vi "Build Application and Installer.vi"(10 "Package Version":string, 11 "Path to project":path) -> (0 "error out":errorcluster)   [LabVIEW 2019]
doc: "Builds the Application (EXE) and Installer with <b>Package Version</b> from build specs in <b>Path to project</b>"
uses:
  Build/Typedefs/Build Spec Type--combo.ctl
  <vilib>/AppBuilder/AB_API_Simple/Set Build Specification Version (path).vi
  <vilib>/AppBuilder/AB_API_Simple/Build (path).vi
  Build/Build.lvlib
  <vilib>/AppBuilder/AB_API_Simple/NI_App_Builder_API.lvlib
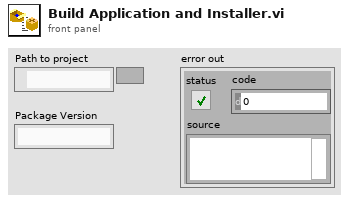
[diagram p1: front panel]
types:
  T1 = typedef "Build.lvlib/Build Spec Type--combo.ctl" = string
  T2 = typedef "Build.lvlib/Build Spec--cluster.ctl" = cluster{"Name":string, "Type":string, "Version":string}
  T3 = typedef "NI_App_Builder_API.lvlib/Build Specification Version.ctl" = cluster{"Major":u16, "Minor":u16, "Fix":u16, "Build":u16}
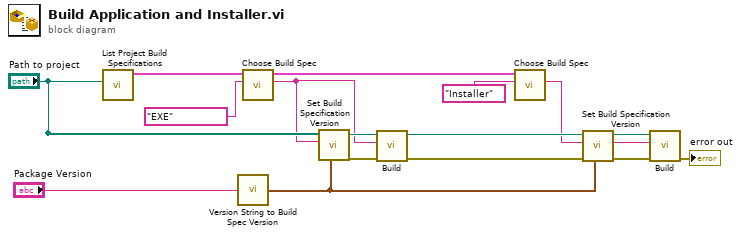
[diagram p0: block diagram]
diagram:
  n1 = call "List Project Build Specifications.vi"("project path"="Path to project") -> ("Build Specs"=w8:T2[])  [unwired: 9 in, 1 out]
  n2 = call "Version String to Build Spec Version.vi"("Package Version"="Package Version") -> ("Build Specification Version"=w2:T3)
  n3 = call "Choose Build Spec.vi"("Build Type"=T1 "EXE", "Build Specs"=w8) -> ("Name"=w7:string, "Build Specs out"=w9:T2[])  [unwired: 6 in, 2 out]
  n4 = call-poly <vilib>:"Set Build Specification Version.vi"("Build Specification Version"=w2, "Name of build specification"=w7, "Path to project"="Path to project") -> ("error out"=w3:errorcluster)  [unwired: 8 in]
  n5 = call-poly <vilib>:"Build.vi"("error in (no error)"=w3, "Name of build specification (if empty: build all)"=w7, "Path to project"="Path to project") -> ("error out"=w4:errorcluster)  [unwired: 7 in, 1 out]
  n6 = call "Choose Build Spec.vi"("Build Type"=T1 "Installer", "Build Specs"=w9) -> ("Name"=w1:string)  [unwired: 6 in, 3 out]
  n7 = call-poly <vilib>:"Set Build Specification Version.vi"("Build Specification Version"=w2, "error in (no error)"=w4, "Name of build specification"=w1, "Path to project"="Path to project") -> ("error out"=w5:errorcluster)  [unwired: 7 in]
  n8 = call-poly <vilib>:"Build.vi"("error in (no error)"=w5, "Name of build specification (if empty: build all)"=w1, "Path to project"="Path to project") -> ("error out"=→"error out":errorcluster)  [unwired: 7 in, 1 out]
